vi "test_TrajectoryRK110428Fiber_Spiral.vi"() -> ()   [LabVIEW 2010, in "TrajectoryRK110428Fiber_Spiral.lvclass"]
uses:
  TrajectoryRK110428Fiber_Spiral.lvclass
  FPGAWrapper/FPGAWrapperRK110512Fiber/FPGAWrapperRK110512Fiber_Spiral/fiber_spiral_parameters.ctl
  common/classes/ErrorController/ErrorController/ErrorController.lvclass
  common/classes/ErrorController/ErrorController/class_data.vi
  FPGAWrapper/FPGAWrapperRK110512Fiber/FPGAWrapperRK110512Fiber_Spiral/FPGAWrapperRK110512Fiber_Spiral.lvclass
panel:
  in  "Fiber spiral parameters":T1={"Fiber Frequency"=2200, "Imaging Periods"=100, "Settling Periods"=50, "Resting Periods"=30, "Amplitude X"=0.5, "Amplitude Y"=0.5, "Phase difference"=90.0, "Initial Amplitude X"=0.0, "Initial Amplitude Y"=0.0} {"Initial Amplitude Y" min=0.0 max=3.0 step=0.1; "Initial Amplitude X" min=0.0 max=3.0 step=0.1; "Phase difference" min=0.0 max=360.0 step=5.0; "Amplitude Y" min=0.0 max=3.0 step=0.1; "Amplitude X" min=0.0 max=3.0 step=0.1}
  in  "Pixel dwell time":dbl
  in  "initialise":bool
  in  "Number of frames":i32
  in  "stop":bool
  in  "startButton":bool
  in  "createButton":bool
  out "error loaded?":bool
  # "Test VI for TrajectoryRK110428Fiber_Spiral"
  # "[µs]"
  # "[Hz]"
  # "[V]"
  # "[V]"
  # "[deg]"
  # "[V]"
  # "[V]"
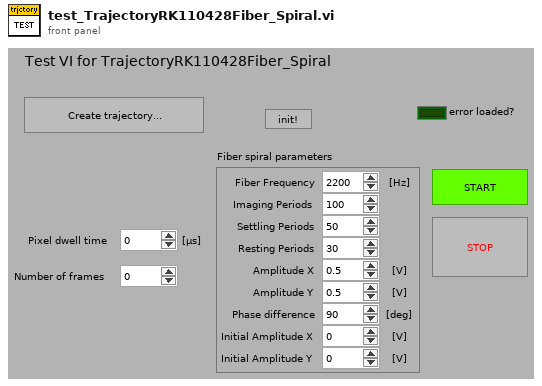
[diagram p1: front panel]
types:
  T1 = typedef "FPGAWrapperRK110512Fiber_Spiral.lvclass/fiber_spiral_parameters.ctl" = cluster{"Fiber Frequency":u16, "Imaging Periods":u16, "Settling Periods":u16, "Resting Periods":u16, "Amplitude X":dbl, "Amplitude Y":dbl, "Phase difference":dbl, "Initial Amplitude X":dbl, "Initial Amplitude Y":dbl}
  T2 = typedef "plugin_specification.ctl" = cluster{"class path":string, "configuration":string, "label":string, "settings name":string}
  T3 = typedef "XComponentSpecification.xctl/data.ctl" = cluster{"class path":string, "configuration":string, "label":string, "settings name":string}
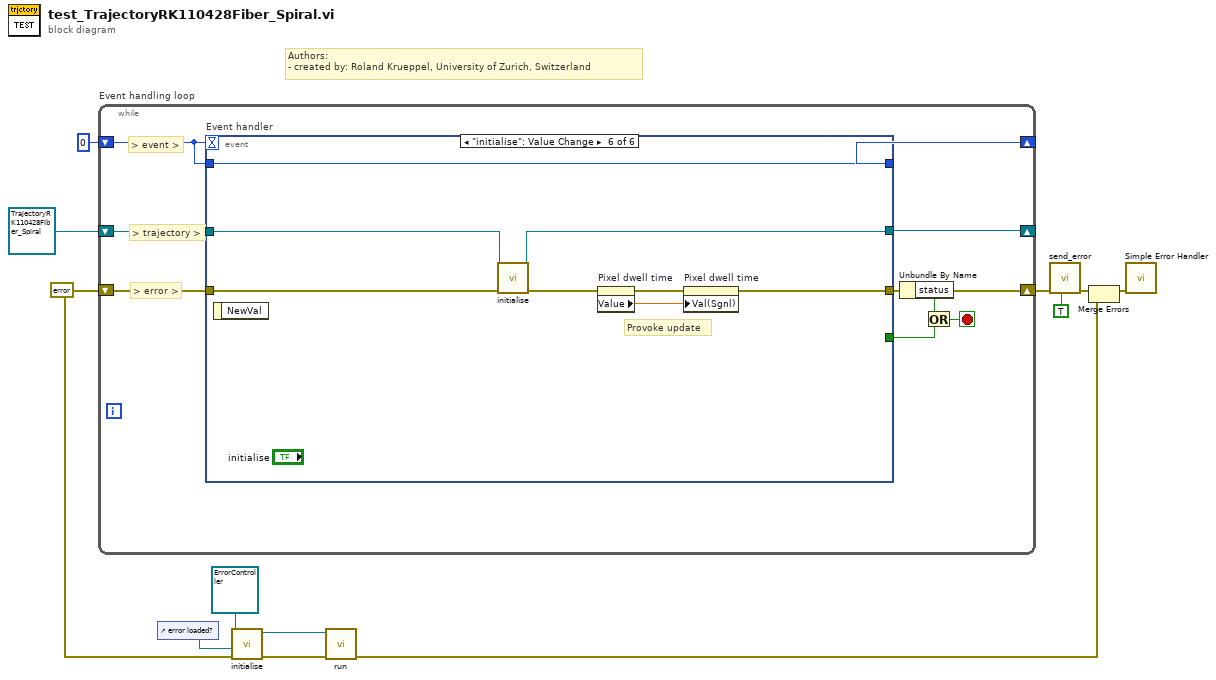
[diagram p0: block diagram]
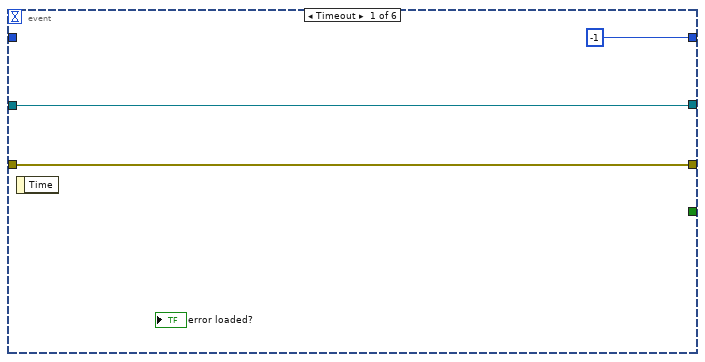
[diagram p2: hidden frame]
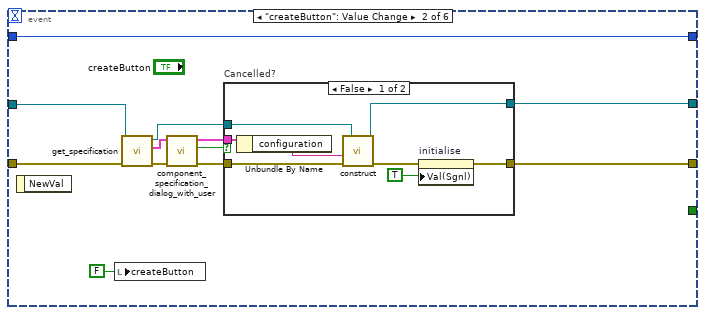
[diagram p3: hidden frame]
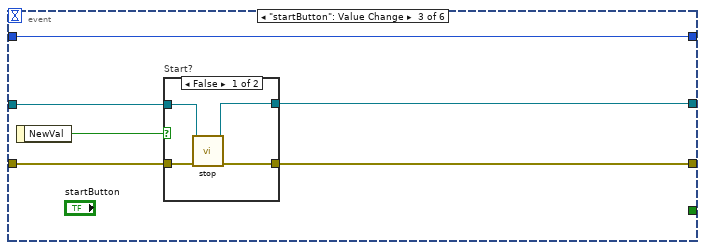
[diagram p5: hidden frame]
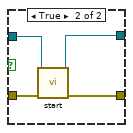
[diagram p6: hidden frame]
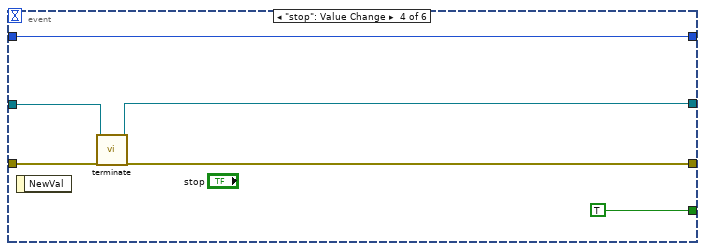
[diagram p7: hidden frame]
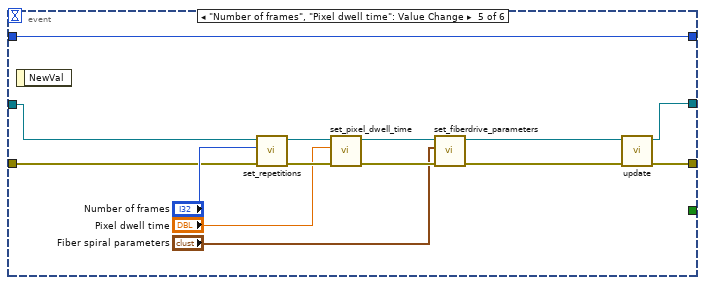
[diagram p8: hidden frame]
diagram:
  w9 = errorcluster {"status"=FALSE, "code"=0, "source"=""} ("error out")
  # "Authors: \n- created by: Roland Krueppel, University of Zurich, Switzerland"
  n1 = while "Event handling loop" {
    shift-right: [w14] -> _
    shift-left: 0 -> [w13]
    shift-right: [w18] -> w4
    shift-left: w9 -> [w21]
    shift-right: [w19] -> _
    shift-left: refnum<class "TrajectoryRK110428Fiber_Spiral.lvclass"> refnum ("TrajectoryRK110428Fiber_Spiral.lvclass") -> [w20]
    stop <- w16 stop-if-true
    # "> trajectory >"
    # "> error >"
    # "> event >"
    n2 = event "Event handler" shown="[5] \"initialise\": Value Change" {
      selector: _ -> [_ _ _ _ _ _]
      dyn-events: _ -> [_ _ _ _ _ _]
      timeout: w13 -> [_ _ _ _ _ _]
      tunnel: [-1 w36 w52 w65 w80 w88] -> w14
      tunnel: w13 -> [_ w36 w52 w65 w80 w88]
      tunnel: [w22 w33 w49 w63 w72 w81] -> w18
      tunnel: w21 -> [w22 w30 w50 w64 w78 w87]
      tunnel: [w23 w34 w48 w61 w73 w85] -> w19
      tunnel: w20 -> [w23 w28 w51 w62 w77 w86]
      tunnel: [_ _ _ TRUE ("stop") _ _] -> w15
      event Timeout {
        n3 = event-data() -> ()  [unwired: 1 in, 1 out]
      }
      event "createButton": Value Change {
        n4 = event-data() -> ()  [unwired: 1 in, 1 out]
        n5 = local write "createButton"(FALSE ("createButton")) -> ()
        n6 = call-dynamic "get_specification.vi"("error in (no error)"=w30, "GenericPlugin in"=w28) -> ("error out"=w31:errorcluster, "component specification"=w32:T2, "GenericPlugin out"=w27:refnum<class "TrajectoryRK110428Fiber_Spiral.lvclass">)  [unwired: 6 in, 1 out]
        n7 = call "component_specification_dialog_with_user.vi"("error in (no error)"=w31, "component specification in"=w32) -> ("error out"=w29:errorcluster, "cancelled?"=w25:bool, "component specification out"=w26:T3)  [unwired: 7 in]
        n8 = case "Cancelled?" shown="False" w25 {
          tunnel: [w44 w45] -> w34
          tunnel: [w41 w46] -> w33
          tunnel: w29 -> [w40 w46]
          tunnel: w27 -> [w39 w45]
          tunnel: w26 -> [w38 _]
          frame False {
            n9 = Unbundle By Name(w38) -> ("configuration"=w37:string)
            n10 = call-dynamic "construct.vi"("error in (no error)"=w40, "configuration name"=w37, "TrajectoryRK110428Fiber in"=w39) -> ("error out"=w42:errorcluster, "TrajectoryRK110428Fiber out"=w44:refnum<class "TrajectoryRK110428Fiber_Spiral.lvclass">)  [unwired: 7 in]
            n11 = property on="initialise" class="Bool (strict)"(error in=w42, "Val(Sgnl)"=TRUE ("Value (Signaling)")) -> (error out=w41:errorcluster)  [unwired: 1 in, 1 out]
          }
          frame True {
          }
        }
      }
      event "startButton": Value Change {
        n12 = event-data() -> ("NewVal"=w47:bool)  [unwired: 1 in]
        n13 = case "Start?" shown="False" w47 {
          tunnel: w51 -> [w54 w60]
          tunnel: w50 -> [w56 w59]
          tunnel: [w55 w58] -> w49
          tunnel: [w53 w57] -> w48
          frame False {
            n14 = call-dynamic "stop.vi"("error in (no error)"=w56, "TrajectoryMG100122GenericFPGA in"=w54) -> ("error out"=w55:errorcluster, "TrajectoryMG100122GenericFPGA out"=w53:refnum<class "TrajectoryRK110428Fiber_Spiral.lvclass">)  [unwired: 8 in]
          }
          frame True {
            n15 = call-dynamic "start.vi"("error in (no error)"=w59, "TrajectoryMG100122GenericFPGA in"=w60) -> ("error out"=w58:errorcluster, "TrajectoryMG100122GenericFPGA out"=w57:refnum<class "TrajectoryRK110428Fiber_Spiral.lvclass">)  [unwired: 8 in]
          }
        }
      }
      event "stop": Value Change {
        n16 = event-data() -> ()  [unwired: 1 in, 1 out]
        n17 = call-dynamic "terminate.vi"("error in (no error)"=w64, "GenericPlugin in"=w62) -> ("error out"=w63:errorcluster, "GenericPlugin out"=w61:refnum<class "TrajectoryRK110428Fiber_Spiral.lvclass">)  [unwired: 8 in]
      }
      event "Number of frames", "Pixel dwell time": Value Change {
        n18 = event-data() -> ()  [unwired: 1 in, 1 out]
        n19 = call-dynamic "set_repetitions.vi"("error in (no error)"=w78, "repetitions"="Number of frames", "GenericTrajectory in"=w77) -> ("error out"=w76:errorcluster, "GenericTrajectory out"=w75:refnum<class "TrajectoryRK110428Fiber_Spiral.lvclass">)  [unwired: 7 in]
        n20 = call-dynamic "set_pixel_dwell_time.vi"("error in (no error)"=w76, "Pixel dwell time"="Pixel dwell time", "TrajectoryRK110428Fiber in"=w75) -> ("error out"=w71:errorcluster, "TrajectoryRK110428Fiber out"=w69:refnum<class "TrajectoryRK110428Fiber_Spiral.lvclass">)  [unwired: 7 in]
        n21 = call-dynamic "set_fiberdrive_parameters.vi"("error in (no error)"=w71, "Fiber spiral parameters"="Fiber spiral parameters", "TrajectoryRK110428Fiber in"=w69) -> ("error out"=w68:errorcluster, "TrajectoryRK110428Fiber out"=w70:refnum<class "TrajectoryRK110428Fiber_Spiral.lvclass">)  [unwired: 7 in]
        n22 = call-dynamic "update.vi"("error in (no error)"=w68, "TrajectoryRK110428Fiber in"=w70) -> ("error out"=w72:errorcluster, "TrajectoryRK110428Fiber out"=w73:refnum<class "TrajectoryRK110428Fiber_Spiral.lvclass">)  [unwired: 8 in]
      }
      event "initialise": Value Change {
        # "Provoke update"
        n23 = event-data() -> ()  [unwired: 1 in, 1 out]
        n24 = call-dynamic "initialise.vi"("error in (no error)"=w87, "GenericPlugin in"=w86) -> ("error out"=w84:errorcluster, "GenericPlugin out"=w85:refnum<class "TrajectoryRK110428Fiber_Spiral.lvclass">)  [unwired: 8 in]
        n25 = property on="Pixel dwell time" class="DigNum (strict)"(error in=w84) -> (error out=w82:errorcluster, "Value"=w83:dbl)  [unwired: 1 in, 1 out]
        n26 = property on="Pixel dwell time" class="DigNum (strict)"(error in=w82, "Val(Sgnl)"=w83) -> (error out=w81:errorcluster)  [unwired: 1 in, 1 out]
      }
    }
    n27 = Unbundle By Name(w18) -> ("status"=w17:bool)
    n28 = Or(x=w17, y=w15) -> (x .or. y?=w16:bool)
  }
  n29 = control-ref of="error loaded?"() -> (w10:refnum<vi>)
  n30 = call-dynamic "initialise.vi"("error in (no error)"=w9, "error boolean"=w10, "ErrorController in"=refnum<class "ErrorController.lvclass"> refnum ("ErrorController.lvclass")) -> ("error out"=w7:errorcluster, "ErrorController out"=w8:refnum<class "ErrorController.lvclass">)  [unwired: 7 in]
  n31 = call "run.vi"("error in (no error)"=w7, "ErrorController in"=w8) -> ("error out"=w3:errorcluster)  [unwired: 8 in, 1 out]
  n32 = call "send_error.vi"("last error? (F)"=TRUE, "error in (no error)"=w4) -> ("error out"=w5:errorcluster)  [unwired: 9 in]
  n33 = Merge Errors(w5, w3) -> (w2:errorcluster)
  n34 = call <vilib>:"Simple Error Handler.vi"("error in (no error)"=w2) -> ()  [unwired: 4 in, 5 out]
